vi "Fetch Power Measurement Sample Statistic Counters.vi"(8 "error in (no error)":errorcluster, 9 "Instance (1)":i32=1, 11 "VISA resource name":refnum<visa-resource-name>) -> (0 "error out":errorcluster, 1 "Sample Count":i32, 2 "Reliability":i32, 3 "VISA resource name out":refnum<visa-resource-name>, 4 "Sample Time":dbl format="%^.3e")   [LabVIEW 2020, in "Rohde&Schwarz CMXP GPRF.lvlib"]
doc: "Returns the sample counters in \"Statistic\" evaluation mode (rscmwgprf Configure Power Measurement Result Mode.vi).\n\nAttribute:\nRSCMXPGPRF_ATTR_FETCH_POWER_MEASUREMENT_SAMPLE_STATISTIC_COUNTERS\n\nRemote-control command:\nFETCh:GPRF:MEAS<i>:POWer:CCDF:SAMPle?"
uses:
  <instrlib>/Rohde&Schwarz CMXP GPRF/Rohde&Schwarz CMXP GPRF.lvlib
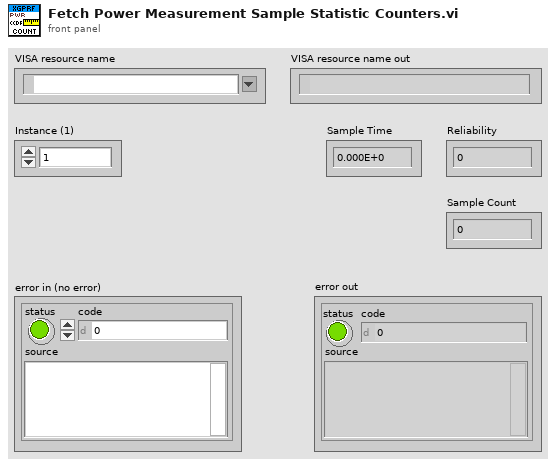
[diagram p1: front panel]
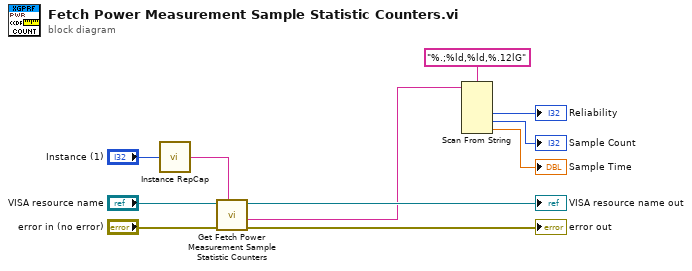
[diagram p0: block diagram]
diagram:
  n1 = call <instrlib>:"Instance RepCap.vi"("Instance in"="Instance (1)") -> ("Instance out"=w6:string)
  n2 = call "Get Fetch Power Measurement Sample Statistic Counters"("Repeated Capabilities"=w6, "error in (no error)"="error in (no error)", "instrument handle"="VISA resource name") -> ("error out"=→"error out":errorcluster, "Fetch Power Measurement Sample Statistic Counters"=w3:string, "instrument handle out"=→"VISA resource name out":refnum<visa-resource-name>)  [unwired: 6 in]
  n3 = Scan From String(format string="%.;%ld,%ld,%.12lG", input string=w3) -> (output 1=→"Reliability":i32, output 2=→"Sample Count":i32, output 3=→"Sample Time":dbl)  [unwired: 5 in, 3 out]
